vi "Read_Timestamp_from_Binary.vi"(8 "error in (no error)":errorcluster, 11 "Binary File path":path) -> (0 "error out":errorcluster, 2 "Number of timestamps":i32, 3 "relative timestamp (ns)":u64[](array[numeric]))   [LabVIEW 2020]
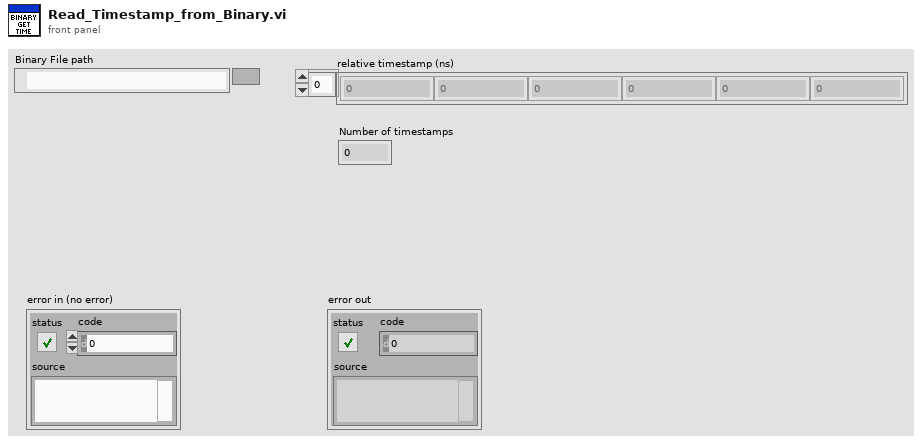
[diagram p1: front panel]
types:
  T1 = enum16{"big-endian, network order", "native, host order", "little-endian"}
  T2 = enum16{"open", "replace", "create", "open or create", "replace or create", "replace or create with confirmation"}
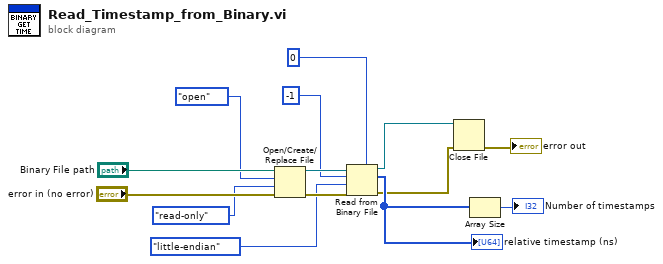
[diagram p0: block diagram]
diagram:
  n1 = Open/Create/Replace File(file path (use dialog)="Binary File path", error in="error in (no error)", operation (0:open)=T2."open", access (0:read/write)=enum16{"read/write", "read-only", "write-only"}."read-only") -> (refnum out=w9:refnum<file>, error out=w8:errorcluster)  [unwired: 2 in, 1 out]
  n2 = Read from Binary File(5:u64 0, 8:w8, 9:T1."little-endian" ("byte order (0:big-endian, network order)"), 10:-1 ("count (1)"), 11:w9) -> (0:w3:errorcluster, 2:w4:u64[], 3:w2:refnum<file>)  [unwired: 1 in, 1 out]
  "relative timestamp (ns)" <- w4
  n3 = Close File(refnum=w2, error in=w3) -> (error out=→"error out":errorcluster)  [unwired: 1 out]
  n4 = Array Size(array=w4) -> (size(s)=→"Number of timestamps":i32)
